vi "xps_panel_DO_set_active_stage.vi"(8 "error in (no error)":errorcluster, 9 "stage_number":i32, 10 "stage_name":string, 11 "newport_xps_panel in":refnum<class "newport_xps_panel.lvclass">) -> (0 "error out":errorcluster, 3 "newport_xps_panel out":refnum<class "newport_xps_panel.lvclass">)   [LabVIEW 2015, in "newport_xps_panel.lvclass"]
uses:
  newport_xps_panel.lvclass
  newport_xps/newport_xps.lvclass
  newport_xps/newport_xps.lvclass/newport_xps.ctl
  UI/panel_class/panel.lvclass
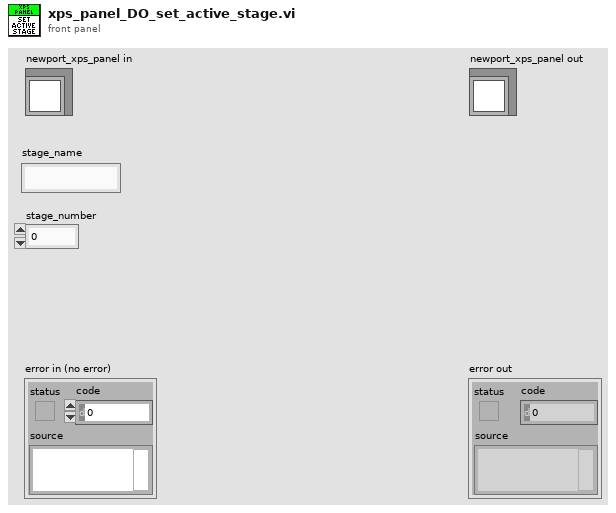
[diagram p1: front panel]
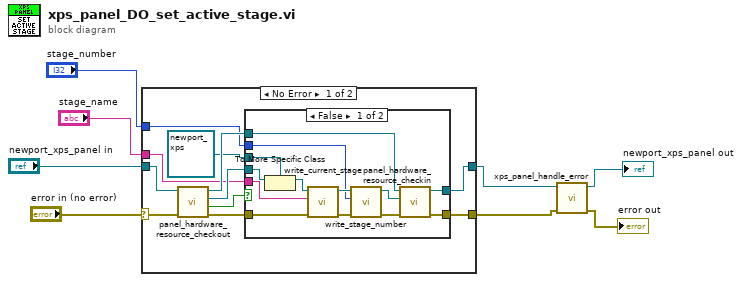
[diagram p0: block diagram]
diagram:
  n1 = case shown="No Error" "error in (no error)" {
    selector: "error in (no error)" -> [w18 w36]
    tunnel: [w13 w36] -> w4
    tunnel: [w12 w35] -> w2
    tunnel: "newport_xps_panel in" -> [w19 w35]
    tunnel: "stage_name" -> [w14 _]
    tunnel: "stage_number" -> [w9 _]
    frame No Error {
      n2 = call "panel_hardware_resource_checkout.vi"("error in (no error)"=w18, "panel in"=w19) -> ("error out"=w11:errorcluster, "timed out?"=w10:bool, "hardware.lvclass"=w15:refnum<class "hardware.lvclass">, "panel out"=w17:refnum<class "newport_xps_panel.lvclass">)  [unwired: 6 in]
      n3 = case shown="False" w10 {
        tunnel: w17 -> [w29 w34]
        tunnel: refnum<class "newport_xps.lvclass"> refnum ("newport_xps.lvclass") -> [w32 _]
        tunnel: w15 -> [w31 _]
        tunnel: w14 -> [w28 _]
        tunnel: [w27 w33] -> w13
        tunnel: [w26 w34] -> w12
        tunnel: w11 -> [w25 w33]
        tunnel: w9 -> [w22 _]
        frame False {
          n4 = To More Specific Class(target class=w32, reference=w31) -> (specific class reference=w30:refnum<class "newport_xps.lvclass">)  [unwired: 1 in, 1 out]
          n5 = call "write_current_stage.vi"("error in (no error)"=w25, "current_stage"=w28, "newport_xps in"=w30) -> ("error out"=w21:errorcluster, "newport_xps out"=w24:refnum<class "newport_xps.lvclass">)  [unwired: 7 in]
          n6 = call "write_stage_number.vi"("error in (no error)"=w21, "stage_number"=w22, "newport_xps in"=w24) -> ("error out"=w20:errorcluster, "newport_xps out"=w23:refnum<class "newport_xps.lvclass">)  [unwired: 7 in]
          n7 = call "panel_hardware_resource_checkin.vi"("error in (no error)"=w20, "hardware.lvclass"=w23, "panel in"=w29) -> ("error out"=w27:errorcluster, "panel out"=w26:refnum<class "newport_xps_panel.lvclass">)  [unwired: 7 in]
        }
        frame True {
        }
      }
    }
    frame Error {
    }
  }
  n8 = call "xps_panel_handle_error.vi"("error in (no error)"=w4, "newport_xps_panel in"=w2) -> ("error out"=→"error out":errorcluster, "newport_xps_panel out"=→"newport_xps_panel out":refnum<class "newport_xps_panel.lvclass">)  [unwired: 8 in]
